vi "TEST_harness_FXP_ss_matmult.vi"() -> ()   [LabVIEW 2019, in "SS_Compensators.lvclass"]
uses:
  SS_Compensators.lvclass
  C:/Program Files (x86)/National Instruments/LabVIEW 2019/vi.lib/addons/_JKI Toolkits/VI Tester/TestCase.llb/TestCase.lvclass
  <vilib>/Utility/file.llb/Read Delimited Spreadsheet (DBL).vi
  <vilib>/rvi/DesktopExecutionNode/Execution/niFpgaDEN_Execute.vi
  <vilib>/rvi/DesktopExecutionNode/DesktopExecutionNode.xnode
  <vilib>/Wiresmith Technology/VITAC (VI Tester Advanced Comparisons)/VITAC.lvlib
panel:
  out "TestCase out":refnum<class "SS_Compensators.lvclass">
  in  "TestCase in":refnum<class "SS_Compensators.lvclass">
  out "Yk":fxp<+/-,36,13>[](array[numeric])
  out "u":dbl[](array[numeric])
  out "y":dbl[](array[numeric])
  out "Waveform Graph":dbl[][](graph)
  out "NS +1":u8=2
  out "ABC_vec":fxp<+/-,32,6>[](array[numeric])
  out "error out":errorcluster
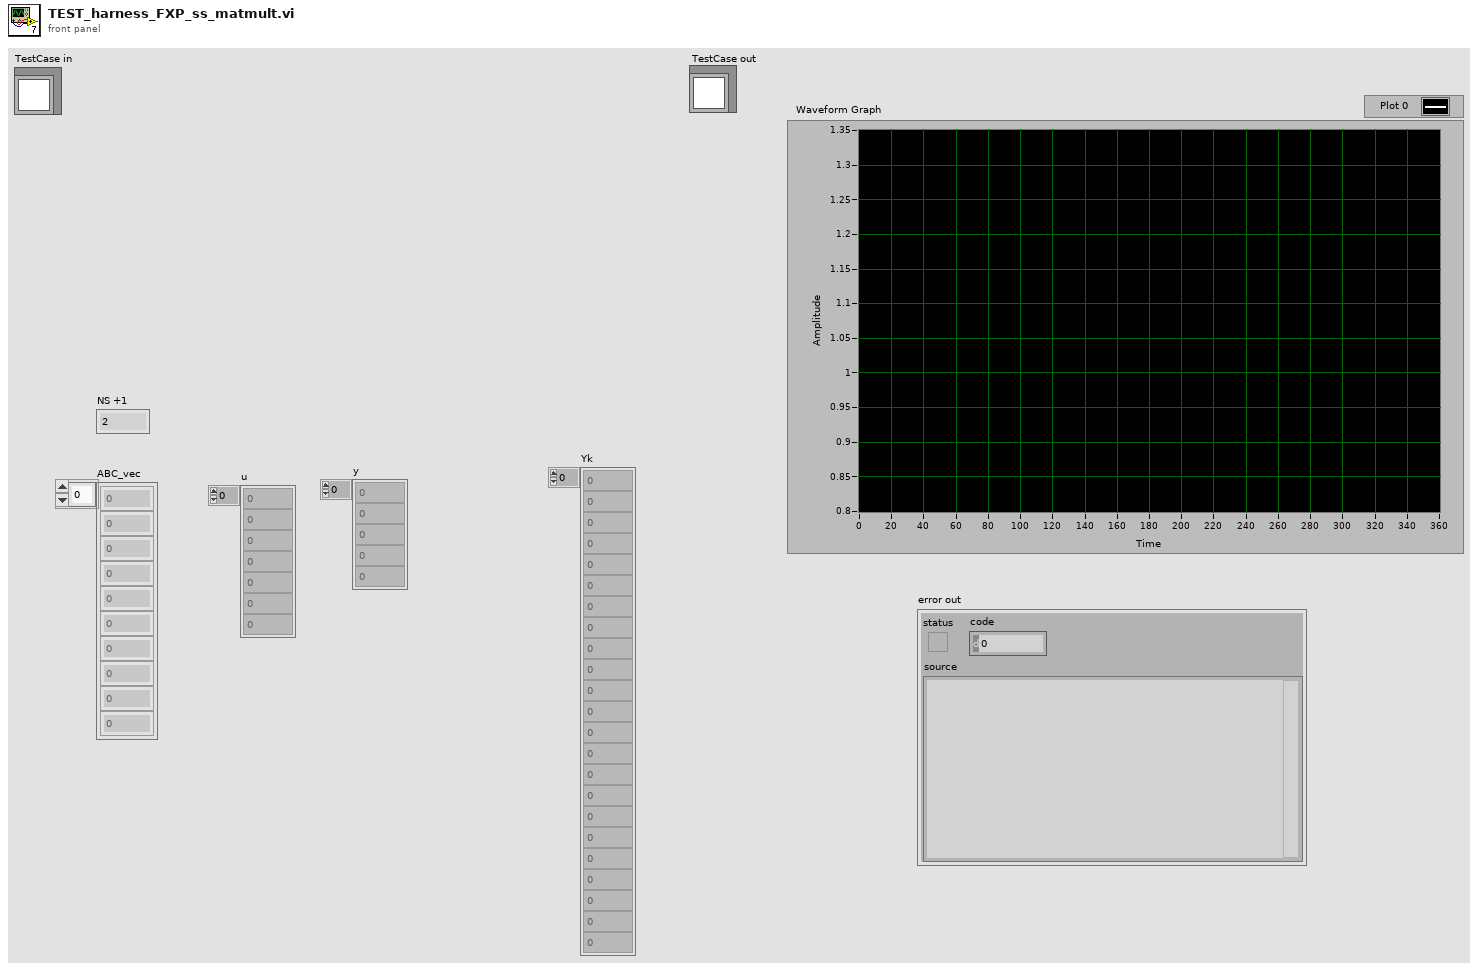
[diagram p1: front panel]
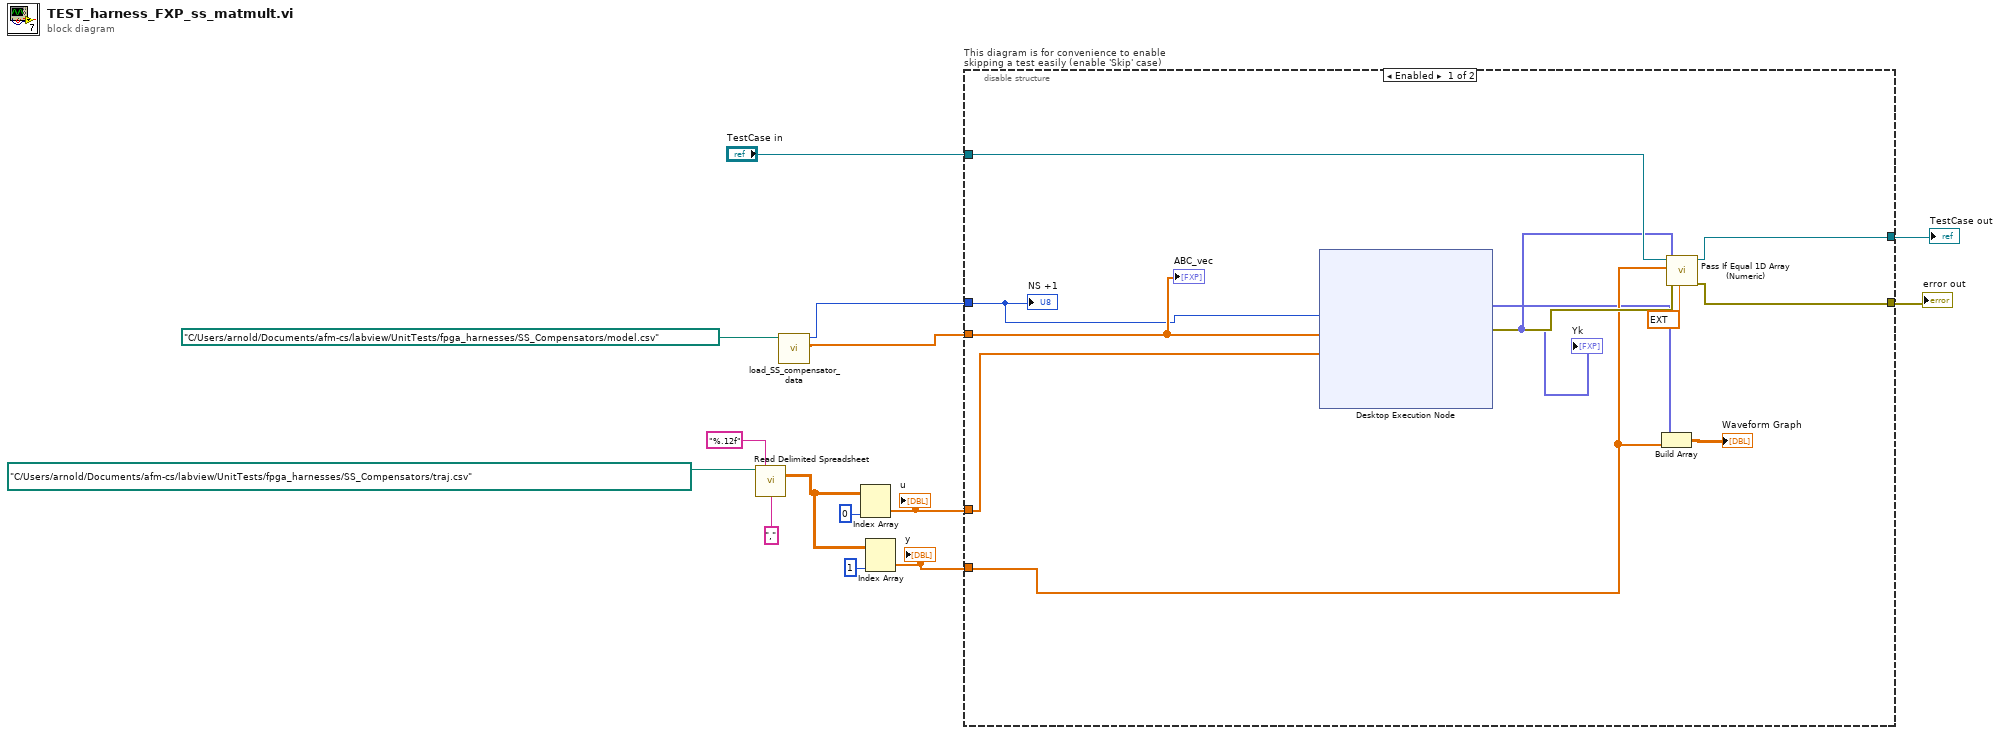
[diagram p0: block diagram]
diagram:
  n1 = call-poly <vilib>:"Read Delimited Spreadsheet.vi"("file path (dialog if empty)"=path "C:/Users/arnold/Documents/afm-cs/labview/UnitTests/fpga_harnesses/SS_Compensators/traj.csv", "format (%.3f)"="%.12f", "delimiter (\\t)"="," ("delimiter (\\t)")) -> ("all rows"=w8:dbl[][])  [unwired: 7 in, 5 out]
  n2 = call "load_SS_compensator_data.vi"("Path"=path "C:/Users/arnold/Documents/afm-cs/labview/UnitTests/fpga_harnesses/SS_Compensators/model.csv") -> ("PHI_col"=w1:dbl[], "Ns_1"=w2:i32)  [unwired: 7 in, 2 out]
  n3 = Index Array(array=w8, index (col)=0 ("disabled index (col)")) -> (element=w7:dbl[])  [unwired: 1 in]
  "u" <- w7
  n4 = Index Array(array=w8, index (col)=1 ("disabled index (col)")) -> (element=w6:dbl[])  [unwired: 1 in]
  "y" <- w6
  n5 = disable-structure "This diagram is for convenience to enable skipping a test easily (enable 'Skip' case)" shown="Enabled" {
    disable-tunnel: [w21 _] -> w14
    disable-tunnel: w7 -> [w23 _]
    disable-tunnel: w6 -> [w18 _]
    disable-tunnel: w1 -> [w24 _]
    disable-tunnel: [w20 w26] -> w5
    disable-tunnel: "TestCase in" -> [w19 w26]
    disable-tunnel: w2 -> [w15 _]
    frame Enabled {
      n6 = xnode "Desktop Execution Node"("Ns_nsw"=w15, "ABCD_col"=w24, "Uk"=w23) -> ("Error Out"=w22:errorcluster, "Yk"=w17:fxp<+/-,36,13>[])  [unwired: 1 in, 1 out]
      "Yk" <- w17
      n7 = Build Array(w17, w18) -> (→"Waveform Graph":dbl[][])
      n8 = call <vilib>:"Pass If Equal 1D Array (Numeric).vi"("delta (optional)"=ext 0.00099999999999999999996, "error in (no error)"=w22, "actual"=w17, "expected"=w18, "TestCase in"=w19) -> ("error out"=w21:errorcluster, "TestCase out"=w20:refnum<class "SS_Compensators.lvclass">)  [unwired: 5 in]
      "NS +1" <- w15
      "ABC_vec" <- w24
    }
    frame Disabled {
      # "skip test result while test is under development"
    }
  }
  "error out" <- w14
  "TestCase out" <- w5
